vi "Exercicio0111.vi"() -> ()   [LabVIEW 2017]
uses:
  <vilib>/MakerHub/LINX/Public/Peripherals/Digital/Digital Write 1 Chan.vi
  <vilib>/MakerHub/LINX/Public/Peripherals/Digital/Digital Read 1 Chan.vi
  <vilib>/MakerHub/LINX/Public/Peripherals/PWM/PWM Set Duty Cycle 1 Chan.vi
  <vilib>/MakerHub/LINX/Public/Peripherals/Digital/Digital Write N Chans.vi
  <vilib>/MakerHub/LINX/Public/Peripherals/Digital/Digital Read N Chans.vi
  <vilib>/MakerHub/LINX/Private/Local IO/LinxDigitalWrite.vi
  <vilib>/MakerHub/LINX/Public/Utilities/Check Channel.vi
  <vilib>/MakerHub/LINX/Private/Local IO/LinxDigitalRead.vi
  <vilib>/MakerHub/LINX/Public/Utilities/Open Serial.vi
  <vilib>/MakerHub/LINX/Private/Utilties/Generate Error.vi
  <vilib>/MakerHub/LINX/Public/Peripherals/PWM/PWM Set Duty Cycle N Chans.vi
  <vilib>/MakerHub/LINX/LMH-LINX.lvlib
panel:
  out "LED verde do protoboard":bool
  out "Status Botão":string
  out "Período (ms)":dbl
  out "Tensão":dbl
  in  "Porta - Arduino":refnum<visa-resource-name>="N/A"
  in  "Frequência (Hz)":dbl(slide) scale=1.0..10.0
  out "LED amarelo \ndo protoboard":bool
  out "Valor do botão\ndo protoboard":bool
  in  "Chave no programa":bool
  in  "Stop":bool
  in  "PWM (%)":dbl(slide) scale=0.0..100.0
  # "Aciona LED vermelho \ndo protoboard"
  # "%"
  # "Aciona LED amarelo \ndo protoboard"
  # "0 V"
  # "1V"
  # "2V"
  # "3V"
  # "4V"
  # "5V"
  # "O botão do protoboard está na \nconfiguração pull up: com o \nbotão não pressionado o LED\n\"Valor do botão do protoboard\"\nserá ligado."
  # "ligado quando \"Chave no programa\"\ne botão do protoboard são acionados"
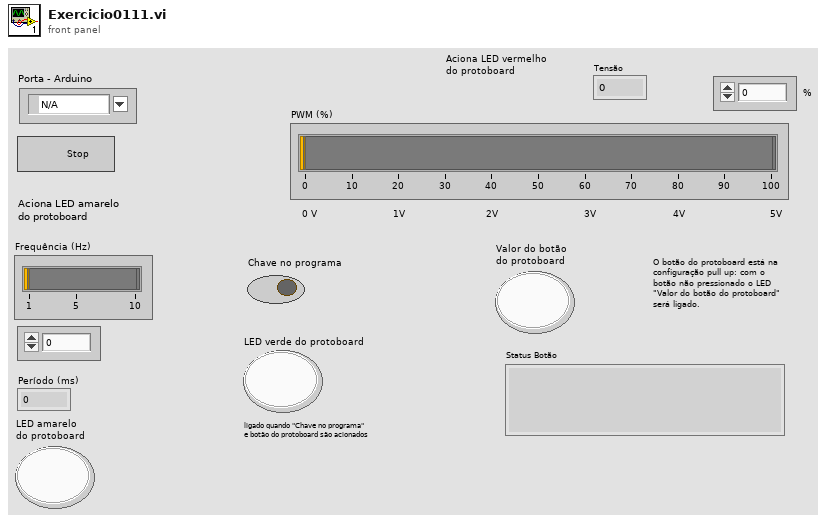
[diagram p1: front panel]
types:
  T1 = typedef "LMH-LINX.lvlib/LINX Ref.ctl" = cluster{"IO":T2, "Interface":T3, "LINX Device Config":T4}
  T2 = typedef "LMH-LINX.lvlib/Platform.ctl" = enum16{"Remote", "Local"}
  T3 = typedef "LMH-LINX.lvlib/Interface.ctl" = enum16{"Serial", "TCP"}
  T4 = typedef "LMH-LINX.lvlib/Device.lvlib/LINX Device Config.ctl" = cluster{"Interface":T3, "COM Port":refnum<visa-resource-name>, "TCP Configuration":T5, "Device Family":u8, "Device ID":u8, "Device Name":string, "TCP Ref":refnum<k5>, "Channels":T6}
  T5 = typedef "LMH-LINX.lvlib/Device.lvlib/TCP Config.ctl" = cluster{"IP Address":string, "Port":u16}
  T6 = typedef "LMH-LINX.lvlib/Channels.ctl" = cluster{"DI":u8[], "DO":u8[], "AI":u8[], "AO":u8[], "PWM":u8[], "QE":u8[], "UART":u8[], "I2C 2":u8[], "SPI":u8[], "CAN":u8[], "Servo":u8[], "AI Ref (V)":dbl, "AI Resolution (Bits)":u8, "AO Ref (V)":dbl, "AO Resolution (Bits)":u8}
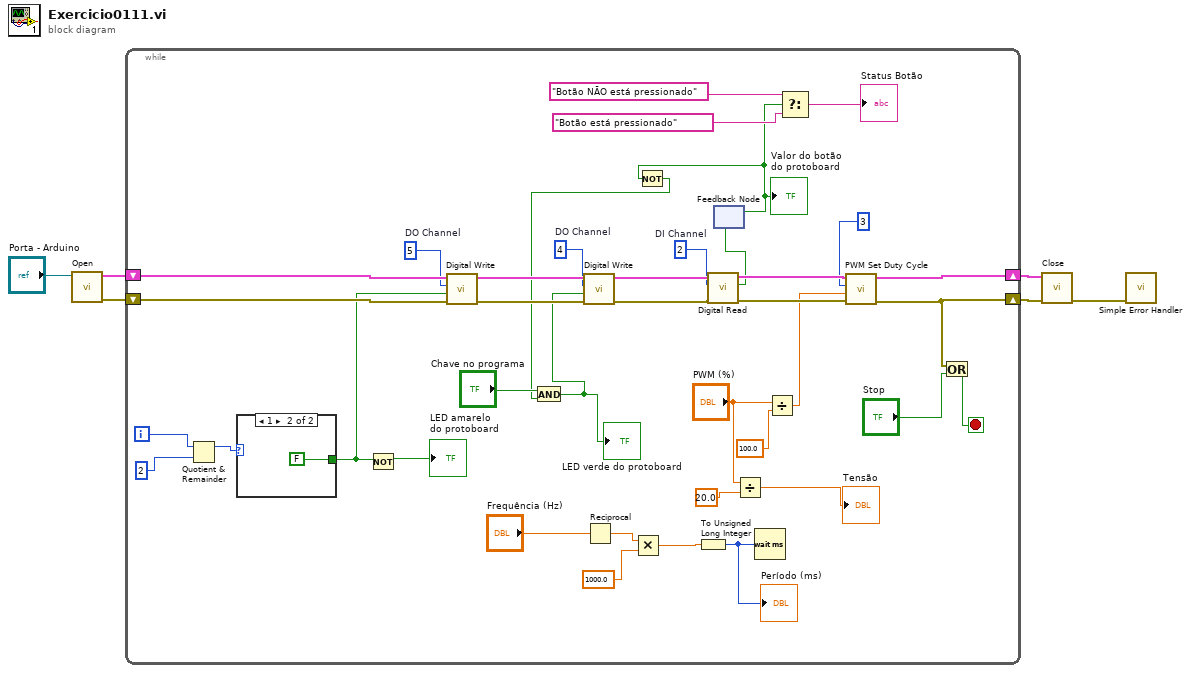
[diagram p0: block diagram]
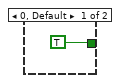
[diagram p2: hidden frame]
diagram:
  n1 = call-poly <vilib>:"Open.vi"("Serial Port"="Porta - Arduino") -> ("Error Out"=w2:errorcluster, "LINX Resource"=w6:T1)  [unwired: 8 in, 1 out]
  n2 = while {
    shift-right: [w43] -> w5
    shift-left: w6 -> [w45]
    shift-right: [w26] -> w3
    shift-left: w2 -> [w41]
    i -> [w23]
    stop <- w24 stop-if-true
    w34 = 2  # DI Channel
    w35 = 4  # DO Channel
    w36 = 5  # DO Channel
    n3 = Quotient & Remainder(x=w23, y=2) -> (x-y*floor(x/y)=w21:i32)  [unwired: 1 out]
    n4 = case shown="1" w21 {
      tunnel: [TRUE FALSE] -> w19
      frame 0, Default {
      }
      frame 1 {
      }
    }
    n5 = Not(x=w19) -> (.not. x?=→"LED amarelo \ndo protoboard":bool)
    n6 = call-poly <vilib>:"Digital Write.vi"("Error In"=w41, "Output Value"=w19, "DO Channel"=w36, "LINX Resource"=w45) -> ("Error Out"=w42:errorcluster, "LINX Resource"=w44:T1)  [unwired: 6 in]
    n7 = Reciprocal(x="Frequência (Hz)") -> (1/x=w31:dbl)
    n8 = Multiply(x=w31, y=1000.0) -> (x*y=w29:dbl)
    n9 = To Unsigned Long Integer(number=w29) -> (unsigned 32bit integer=w15:u32)
    "Período (ms)" <- w15
    n10 = feedback #1() -> (w8:bool)  [unwired: 1 in]
    "Valor do botão\ndo protoboard" <- w8
    n11 = Not(x=w8) -> (.not. x?=w7:bool)
    n12 = And(x="Chave no programa", y=w7) -> (x .and. y?=w11:bool)
    "LED verde do protoboard" <- w11
    n13 = call-poly <vilib>:"Digital Write.vi"("Error In"=w42, "Output Value"=w11, "DO Channel"=w35, "LINX Resource"=w44) -> ("Error Out"=w38:errorcluster, "LINX Resource"=w40:T1)  [unwired: 6 in]
    n14 = call-poly <vilib>:"Digital Read.vi"("Error In"=w38, "DI Channel"=w34, "LINX Resource"=w40) -> ("Error Out"=w37:errorcluster, "DI Value"=w9:bool, "LINX Resource"=w39:T1)  [unwired: 6 in]
    n15 = feedback-in #1(w9) -> ()
    n16 = Divide(x="PWM (%)", y=20.0) -> (x/y=→"Tensão":dbl)
    n17 = Wait (ms)(milliseconds to wait=w15) -> ()  [unwired: 1 out]
    n18 = Divide(x="PWM (%)", y=100.0) -> (x/y=w27:dbl)
    n19 = Select(t="Botão NÃO está pressionado", s=w8, f="Botão está pressionado") -> (s? t:f=→"Status Botão":string)
    n20 = call-poly <vilib>:"PWM Set Duty Cycle.vi"("Error In"=w37, "Duty Cycle (0-1)"=w27, "PWM Channel"=3, "LINX Resource"=w39) -> ("Error Out"=w26:errorcluster, "LINX Resource"=w43:T1)  [unwired: 6 in]
    n21 = Or(x=w26, y="Stop") -> (x .or. y?=w24:bool)
  }
  n22 = call <vilib>:"Close.vi"("Error In"=w3, "LINX Resource"=w5) -> ("Error Out"=w4:errorcluster)  [unwired: 9 in]
  n23 = call <vilib>:"Simple Error Handler.vi"("error in (no error)"=w4) -> ()  [unwired: 4 in, 5 out]
